vi "Create motor.vi"(7 "name":string, 8 "error in (no error)":errorcluster, 9 "StateManager":refnum<class "StateManager.lvclass">, 10 "MotorSim":refnum<class "MotorSim.lvclass">, 11 "Motor in":refnum<class "Motor.lvclass">) -> (0 "error out":errorcluster, 3 "Motor out":refnum<class "Motor.lvclass">)   [LabVIEW 2018, in "Motor.lvclass"]
uses:
  Motor.lvclass
  MotorSim/MotorSim.lvclass
  StateManager/StateManager.lvclass
  Motor.lvclass/Motor.ctl
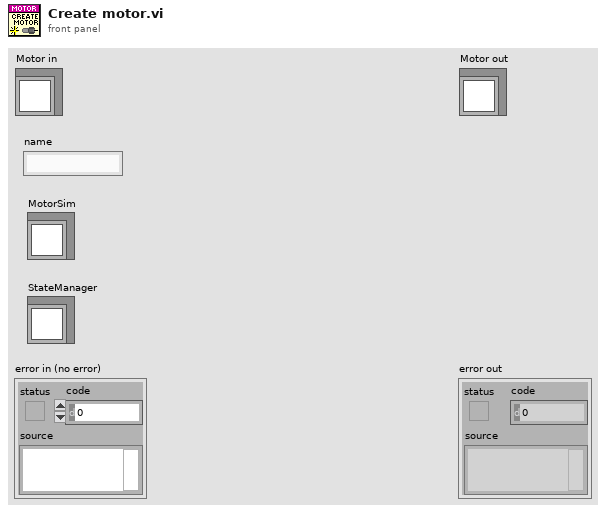
[diagram p1: front panel]
types:
  T1 = cluster{"mode":string, "condition":string, "position":string, "pos_name":string, "pos_id":string}
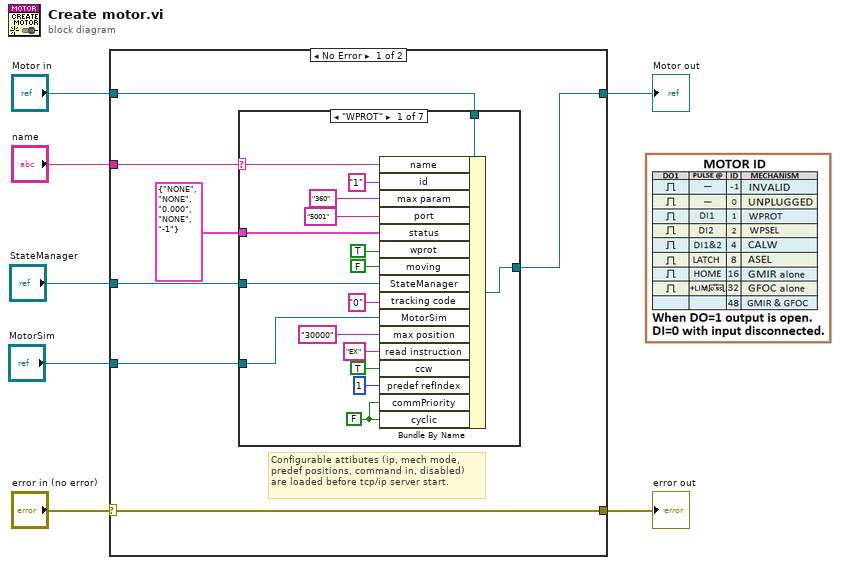
[diagram p0: block diagram]
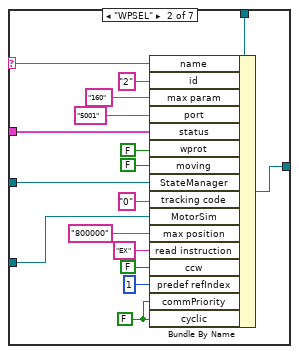
[diagram p2: hidden frame]
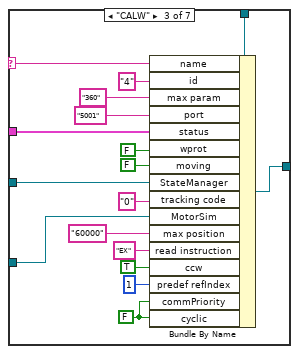
[diagram p3: hidden frame]
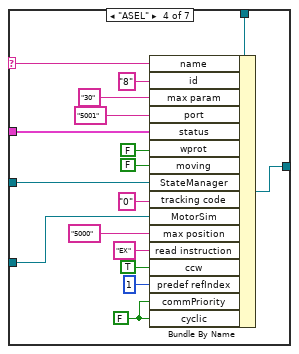
[diagram p4: hidden frame]
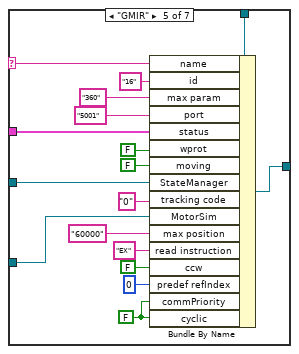
[diagram p5: hidden frame]
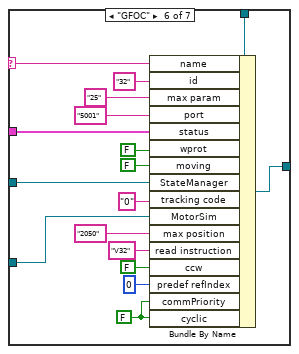
[diagram p6: hidden frame]
diagram:
  n1 = case shown="No Error" "error in (no error)" {
    selector: "error in (no error)" -> [w8 w118]
    tunnel: [w8 w118] -> w6
    tunnel: [w9 w119] -> w4
    tunnel: "Motor in" -> [w10 w119]
    tunnel: "name" -> [w14 _]
    tunnel: "MotorSim" -> [w12 _]
    tunnel: "StateManager" -> [w11 _]
    frame No Error {
      # "Configurable attibutes (ip, mech mode,\npredef positions, command in, disabled)\nare loaded before tcp/ip server start."
      n2 = case shown="\"WPROT\"" w14 {
        selector: w14 -> [w31 w48 w65 w82 w99 w116 _]
        tunnel: T1 {"mode"="NONE", "condition"="NONE", "position"="0.000", "pos_name"="NONE", "pos_id"="-1"} ("status") -> [w30 w47 w64 w81 w98 w115 _]
        tunnel: w12 -> [w29 w46 w63 w80 w97 w114 _]
        tunnel: w11 -> [w28 w45 w62 w79 w96 w113 _]
        tunnel: w10 -> [w18 w35 w52 w69 w86 w103 w117]
        tunnel: [w17 w34 w51 w68 w85 w102 w117] -> w9
        frame "WPROT" {
          w15 = FALSE
          n3 = Bundle By Name(cluster=w18, "name"=w31, "id"="1", "max param"="360", "port"="5001", "status"=w30, "wprot"=TRUE, "moving"=FALSE, "StateManager"=w28, "tracking code"="0", "MotorSim"=w29, "max position"="30000", "read instruction"="EX", "ccw"=TRUE, "predef refIndex"=1, "commPriority"=w15, "cyclic"=w15) -> (w17:refnum<class "Motor.lvclass">)
        }
        frame "WPSEL" {
          w32 = FALSE
          n4 = Bundle By Name(cluster=w35, "name"=w48, "id"="2", "max param"="160", "port"="5001", "status"=w47, "wprot"=FALSE, "moving"=FALSE, "StateManager"=w45, "tracking code"="0", "MotorSim"=w46, "max position"="800000", "read instruction"="EX", "ccw"=FALSE, "predef refIndex"=1, "commPriority"=w32, "cyclic"=w32) -> (w34:refnum<class "Motor.lvclass">)
        }
        frame "CALW" {
          w49 = FALSE
          n5 = Bundle By Name(cluster=w52, "name"=w65, "id"="4", "max param"="360", "port"="5001", "status"=w64, "wprot"=FALSE, "moving"=FALSE, "StateManager"=w62, "tracking code"="0", "MotorSim"=w63, "max position"="60000", "read instruction"="EX", "ccw"=TRUE, "predef refIndex"=1, "commPriority"=w49, "cyclic"=w49) -> (w51:refnum<class "Motor.lvclass">)
        }
        frame "ASEL" {
          w66 = FALSE
          n6 = Bundle By Name(cluster=w69, "name"=w82, "id"="8", "max param"="30", "port"="5001", "status"=w81, "wprot"=FALSE, "moving"=FALSE, "StateManager"=w79, "tracking code"="0", "MotorSim"=w80, "max position"="5000", "read instruction"="EX", "ccw"=TRUE, "predef refIndex"=1, "commPriority"=w66, "cyclic"=w66) -> (w68:refnum<class "Motor.lvclass">)
        }
        frame "GMIR" {
          w83 = FALSE
          n7 = Bundle By Name(cluster=w86, "name"=w99, "id"="16", "max param"="360", "port"="5001", "status"=w98, "wprot"=FALSE, "moving"=FALSE, "StateManager"=w96, "tracking code"="0", "MotorSim"=w97, "max position"="60000", "read instruction"="EX", "ccw"=FALSE, "predef refIndex"=0, "commPriority"=w83, "cyclic"=w83) -> (w85:refnum<class "Motor.lvclass">)
        }
        frame "GFOC" {
          w100 = FALSE
          n8 = Bundle By Name(cluster=w103, "name"=w116, "id"="32", "max param"="25", "port"="5001", "status"=w115, "wprot"=FALSE, "moving"=FALSE, "StateManager"=w113, "tracking code"="0", "MotorSim"=w114, "max position"="2050", "read instruction"="V32", "ccw"=FALSE, "predef refIndex"=0, "commPriority"=w100, "cyclic"=w100) -> (w102:refnum<class "Motor.lvclass">)
        }
        frame "", Default {
        }
      }
    }
    frame Error {
    }
  }
  "error out" <- w6
  "Motor out" <- w4
